vi "InitializeConnection.vi"(8 "error in":errorcluster, 11 "StellarNetSpecAcquisition in":refnum<class "StellarNetSpecAcquisition.lvclass">) -> (0 "error out":errorcluster, 3 "StellarNetSpecAcquisition out":refnum<class "StellarNetSpecAcquisition.lvclass">)   [LabVIEW 2020, in "StellarNetSpecAcquisition.lvclass"]
doc: "Initialize the connection to the driver dll"
uses:
  StellarNetSpecAcquisition.lvclass
  StellarNetSpectrometer.lvclass
  Swdll.dll
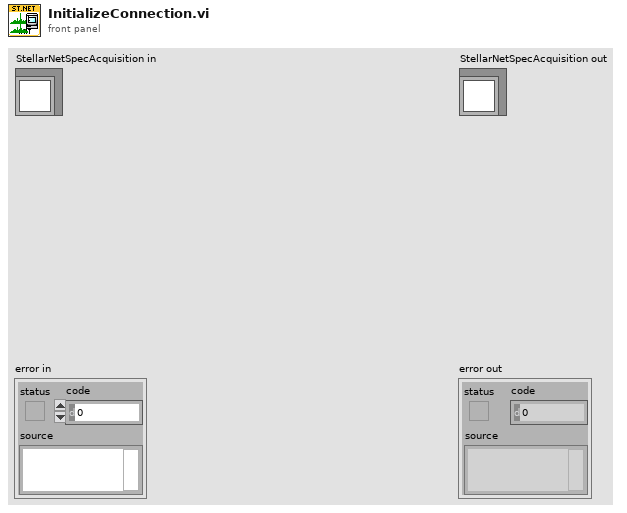
[diagram p1: front panel]
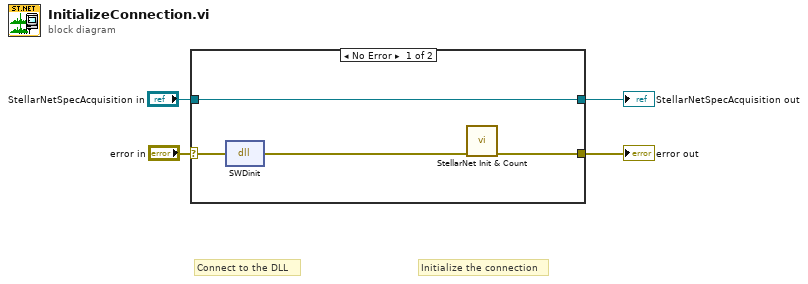
[diagram p0: block diagram]
diagram:
  # "Initialize the connection"
  # "Connect to the DLL"
  n1 = case shown="No Error" "error in" {
    selector: "error in" -> [w6 w10]
    tunnel: [w7 w10] -> w4
    tunnel: [w8 w9] -> w2
    tunnel: "StellarNetSpecAcquisition in" -> [w8 w9]
    frame No Error {
      n2 = dll-call lib="C:/GEECS/Developers Version/source/Device Drivers/StellarNet Black-Comet Spec/SupportLib/StellarNetSpectrometerClass/CommMethods/swdll.dll" fn="SWDinit" label="init"(error in=w6) -> (error out=w5:errorcluster)  [unwired: 3 in, 1 out]
      n3 = call "StellarNet Init & Count.vi"("error in"=w5) -> ("error out"=w7:errorcluster)  [unwired: 9 in, 1 out]
    }
    frame Error {
    }
  }
  "error out" <- w4
  "StellarNetSpecAcquisition out" <- w2
